vi "Main.vi"(8 "error in":errorcluster, 11 "_Rename in":refnum<class "_Rename.lvclass">) -> (0 "error out":errorcluster, 3 "_Rename out":refnum<class "_Rename.lvclass">)   [LabVIEW 2020, in "_Rename.lvlib" / "_Rename.lvclass"]
uses:
  _Rename.lvclass
  _Rename.lvclass/_Rename.ctl
  _Shared/Project Stuff/Project Stuff.lvclass
  _Shared/Name Specs/Name Specs.lvclass
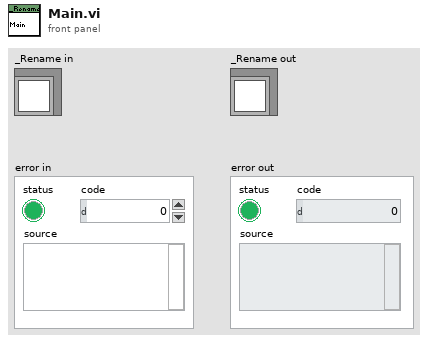
[diagram p1: front panel]
types:
  T1 = typedef "_Shared.lvlib/Name Stuff.ctl" = cluster{"Type (Enum)":T2, "Type (String)":string, "Name Library File Path":path, "Name":string, "Name Type":string}
  T2 = typedef "_Shared.lvlib/Type.ctl" = enum16{"Actor", "Msg"}
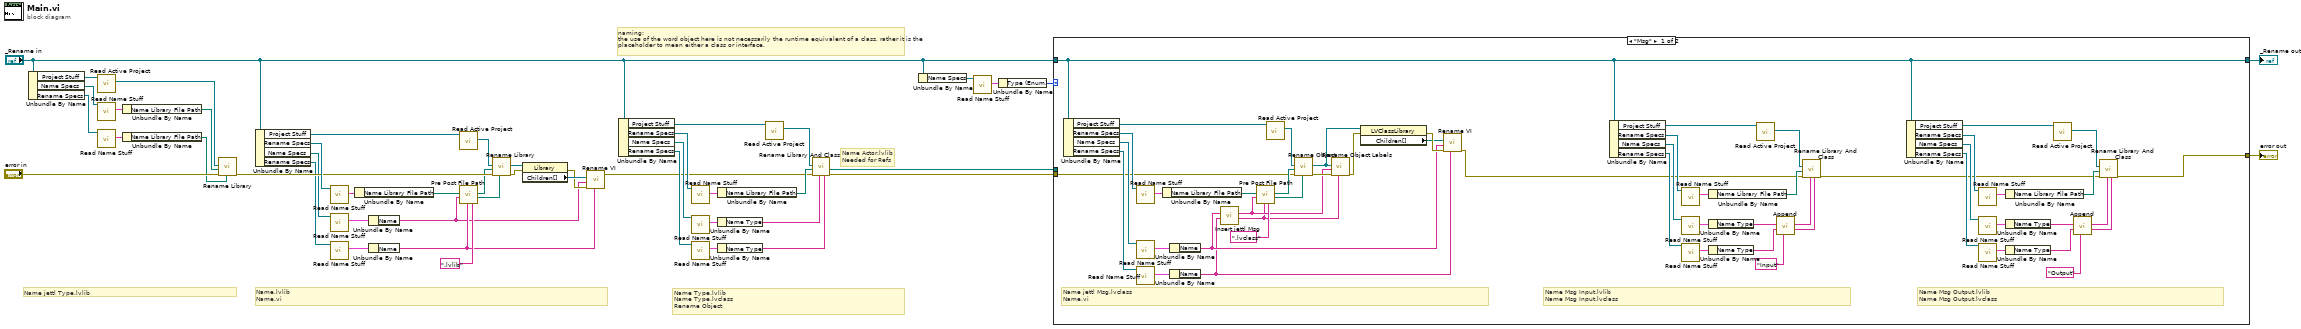
[diagram p0: block diagram]
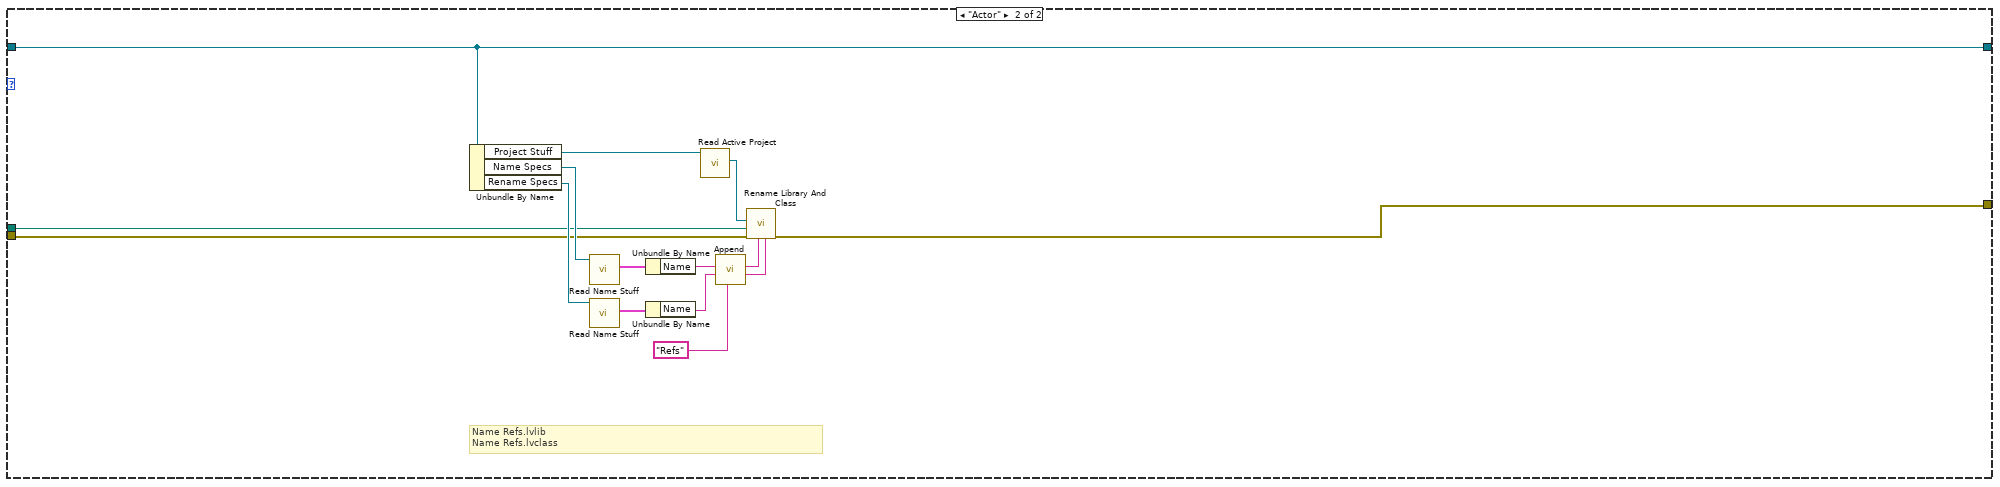
[diagram p2: hidden frame]
diagram:
  # "Name Actor.lvlib\nNeeded for Refs"
  # "Name Type.lvlib\nName Type.lvclass\nRename Object"
  # "naming:\nthe use of the word object here is not necessarily the runtime equivalent of a class, rather it is the placeholder to mean either a class or interface."
  # "Name.lvlib\nName.vi"
  # "Name jettl Type.lvlib"
  n1 = Unbundle By Name("_Rename in") -> ("Project Stuff"=w43:refnum<class "Project Stuff.lvclass">, "Name Specs"=w42:refnum<class "Name Specs.lvclass">, "Rename Specs"=w39:refnum<class "Name Specs.lvclass">)
  n2 = call "Read Active Project.vi"("Project Stuff in"=w43) -> ("Active Project"=w45:refnum<vi>)  [unwired: 10 in]
  n3 = call "Read Name Stuff.vi"("Name Specs in"=w42) -> ("Name Stuff"=w41:T1)  [unwired: 10 in]
  n4 = call "Read Name Stuff.vi"("Name Specs in"=w39) -> ("Name Stuff"=w40:T1)  [unwired: 10 in]
  n5 = Unbundle By Name(w41) -> ("Name Library File Path"=w37:path)
  n6 = Unbundle By Name(w40) -> ("Name Library File Path"=w38:path)
  n7 = call "Rename Library.vi"("Rename Library File Path"=w38, "error in"="error in", "Name Library File Path"=w37, "Active Project"=w45) -> ("error out"=w23:errorcluster)  [unwired: 6 in, 1 out]
  n8 = Unbundle By Name("_Rename in") -> ("Project Stuff"=w25:refnum<class "Project Stuff.lvclass">, "Rename Specs"=w27:refnum<class "Name Specs.lvclass">, "Name Specs"=w21:refnum<class "Name Specs.lvclass">, "Rename Specs"=w18:refnum<class "Name Specs.lvclass">)
  n9 = call "Read Name Stuff.vi"("Name Specs in"=w27) -> ("Name Stuff"=w26:T1)  [unwired: 10 in]
  n10 = call "Read Name Stuff.vi"("Name Specs in"=w21) -> ("Name Stuff"=w20:T1)  [unwired: 10 in]
  n11 = call "Read Name Stuff.vi"("Name Specs in"=w18) -> ("Name Stuff"=w19:T1)  [unwired: 10 in]
  n12 = Unbundle By Name(w26) -> ("Name Library File Path"=w10:path)
  n13 = Unbundle By Name(w20) -> ("Name"=w11:string)
  n14 = Unbundle By Name(w19) -> ("Name"=w12:string)
  n15 = call "Read Active Project.vi"("Project Stuff in"=w25) -> ("Active Project"=w24:refnum<vi>)  [unwired: 10 in]
  n16 = call "Pre Post File Path.vi"("Extension"=".lvlib" ("string"), "Post"=w12, "Pre"=w11, "Rename Library File Path"=w10) -> ("Post File Path"=w8:path, "Pre File Path"=w9:path)  [unwired: 6 in]
  n17 = call "Rename Library.vi"("Rename Library File Path"=w8, "error in"=w23, "Name Library File Path"=w9, "Active Project"=w24) -> ("error out"=w15:errorcluster, "Library Ref"=w17:refnum<vi>)  [unwired: 6 in]
  n18 = property class="Library"(reference=w17, error in=w15) -> (error out=w14:errorcluster, "Children[]"=w16:refnum<vi>[])  [unwired: 1 out]
  n19 = call "Rename VI.vi"("Rename"=w12, "error in"=w14, "VI Name"=w11, "Owned Items[]"=w16) -> ("error out"=w3:errorcluster)  [unwired: 7 in]
  n20 = Unbundle By Name("_Rename in") -> ("Project Stuff"=w44:refnum<class "Project Stuff.lvclass">, "Rename Specs"=w28:refnum<class "Name Specs.lvclass">, "Name Specs"=w29:refnum<class "Name Specs.lvclass">, "Rename Specs"=w30:refnum<class "Name Specs.lvclass">)
  n21 = call "Read Name Stuff.vi"("Name Specs in"=w28) -> ("Name Stuff"=w31:T1)  [unwired: 10 in]
  n22 = call "Read Name Stuff.vi"("Name Specs in"=w29) -> ("Name Stuff"=w33:T1)  [unwired: 10 in]
  n23 = call "Read Name Stuff.vi"("Name Specs in"=w30) -> ("Name Stuff"=w32:T1)  [unwired: 10 in]
  n24 = Unbundle By Name(w31) -> ("Name Library File Path"=w4:path)
  n25 = Unbundle By Name(w33) -> ("Name Type"=w2:string)
  n26 = Unbundle By Name(w32) -> ("Name Type"=w1:string)
  n27 = call "Read Active Project.vi"("Project Stuff in"=w44) -> ("Active Project"=w5:refnum<vi>)  [unwired: 10 in]
  n28 = call "Rename Library And Class.vi"("Post"=w1, "Pre"=w2, "error in"=w3, "Rename Library File Path"=w4, "Active Project"=w5) -> ("error out"=w7:errorcluster, "Intermediate Library File Path"=w6:path)  [unwired: 5 in]
  n29 = Unbundle By Name("_Rename in") -> ("Name Specs"=w34:refnum<class "Name Specs.lvclass">)
  n30 = call "Read Name Stuff.vi"("Name Specs in"=w34) -> ("Name Stuff"=w36:T1)  [unwired: 10 in]
  n31 = Unbundle By Name(w36) -> ("Type (Enum)"=w35:T2)
  n32 = case shown="\"Msg\"" w35 {
    tunnel: w7 -> [w89 w108]
    tunnel: [w53 w103] -> w47
    tunnel: [w55 w112] -> w48
    tunnel: "_Rename in" -> [w55 w112]
    tunnel: w6 -> [_ w106]
    frame "Msg" {
      # "Name Msg Input.lvlib\nName Msg Input.lvclass"
      # "Name Msg Output.lvlib\nName Msg Output.lvclass"
      # "Name jettl Msg.lvclass\nName.vi"
      n33 = Unbundle By Name(w55) -> ("Project Stuff"=w100:refnum<class "Project Stuff.lvclass">, "Rename Specs"=w90:refnum<class "Name Specs.lvclass">, "Name Specs"=w91:refnum<class "Name Specs.lvclass">, "Rename Specs"=w92:refnum<class "Name Specs.lvclass">)
      n34 = call "Read Name Stuff.vi"("Name Specs in"=w90) -> ("Name Stuff"=w94:T1)  [unwired: 10 in]
      n35 = call "Read Name Stuff.vi"("Name Specs in"=w91) -> ("Name Stuff"=w96:T1)  [unwired: 10 in]
      n36 = call "Read Name Stuff.vi"("Name Specs in"=w92) -> ("Name Stuff"=w95:T1)  [unwired: 10 in]
      n37 = Unbundle By Name(w94) -> ("Name Library File Path"=w93:path)
      n38 = Unbundle By Name(w96) -> ("Name"=w52:string)
      n39 = Unbundle By Name(w95) -> ("Name"=w51:string)
      n40 = call "Insert jettl Msg.vi"("Rename"=w51, "Name"=w52) -> ("Post"=w49:string, "Pre"=w50:string)  [unwired: 8 in]
      n41 = call "Pre Post File Path.vi"("Extension"=".lvclass", "Post"=w49, "Pre"=w50, "Rename Library File Path"=w93) -> ("Post File Path"=w98:path, "Pre File Path"=w97:path)  [unwired: 6 in]
      n42 = call "Read Active Project.vi"("Project Stuff in"=w100) -> ("Active Project"=w99:refnum<vi>)  [unwired: 10 in]
      n43 = call "Rename Object.vi"("Post Object File Path"=w98, "error in"=w89, "Pre Object File Path"=w97, "Active Project"=w99) -> ("error out"=w101:errorcluster, "Object Ref"=w88:refnum<vi>)  [unwired: 6 in]
      n44 = call "Rename Object Labels.vi"("Post"=w49, "error in"=w101, "Pre"=w50, "Class Ref"=w88) -> ("error out"=w87:errorcluster)  [unwired: 7 in]
      n45 = property class="LVClassLibrary"(reference=w88, error in=w87) -> (error out=w102:errorcluster, "Children[]"=w86:refnum<vi>[])  [unwired: 1 out]
      n46 = call "Rename VI.vi"("Rename"=w51, "error in"=w102, "VI Name"=w52, "Owned Items[]"=w86) -> ("error out"=w70:errorcluster)  [unwired: 7 in]
      n47 = Unbundle By Name(w55) -> ("Project Stuff"=w84:refnum<class "Project Stuff.lvclass">, "Rename Specs"=w78:refnum<class "Name Specs.lvclass">, "Name Specs"=w79:refnum<class "Name Specs.lvclass">, "Rename Specs"=w80:refnum<class "Name Specs.lvclass">)
      n48 = call "Read Name Stuff.vi"("Name Specs in"=w78) -> ("Name Stuff"=w81:T1)  [unwired: 10 in]
      n49 = call "Read Name Stuff.vi"("Name Specs in"=w79) -> ("Name Stuff"=w83:T1)  [unwired: 10 in]
      n50 = call "Read Name Stuff.vi"("Name Specs in"=w80) -> ("Name Stuff"=w82:T1)  [unwired: 10 in]
      n51 = Unbundle By Name(w81) -> ("Name Library File Path"=w76:path)
      n52 = Unbundle By Name(w83) -> ("Name Type"=w75:string)
      n53 = Unbundle By Name(w82) -> ("Name Type"=w74:string)
      n54 = call "Read Active Project.vi"("Project Stuff in"=w84) -> ("Active Project"=w77:refnum<vi>)  [unwired: 10 in]
      n55 = call "Append.vi"("Append"="Input", "Rename Suffix"=w74, "Name Suffix"=w75) -> ("Post"=w73:string, "Pre"=w72:string)  [unwired: 7 in]
      n56 = call "Rename Library And Class.vi"("Post"=w73, "Pre"=w72, "error in"=w70, "Rename Library File Path"=w76, "Active Project"=w77) -> ("error out"=w54:errorcluster)  [unwired: 5 in, 1 out]
      n57 = Unbundle By Name(w55) -> ("Project Stuff"=w69:refnum<class "Project Stuff.lvclass">, "Rename Specs"=w63:refnum<class "Name Specs.lvclass">, "Name Specs"=w64:refnum<class "Name Specs.lvclass">, "Rename Specs"=w65:refnum<class "Name Specs.lvclass">)
      n58 = call "Read Name Stuff.vi"("Name Specs in"=w63) -> ("Name Stuff"=w66:T1)  [unwired: 10 in]
      n59 = call "Read Name Stuff.vi"("Name Specs in"=w64) -> ("Name Stuff"=w68:T1)  [unwired: 10 in]
      n60 = call "Read Name Stuff.vi"("Name Specs in"=w65) -> ("Name Stuff"=w67:T1)  [unwired: 10 in]
      n61 = Unbundle By Name(w66) -> ("Name Library File Path"=w61:path)
      n62 = Unbundle By Name(w68) -> ("Name Type"=w60:string)
      n63 = Unbundle By Name(w67) -> ("Name Type"=w59:string)
      n64 = call "Read Active Project.vi"("Project Stuff in"=w69) -> ("Active Project"=w62:refnum<vi>)  [unwired: 10 in]
      n65 = call "Append.vi"("Append"="Output", "Rename Suffix"=w59, "Name Suffix"=w60) -> ("Post"=w58:string, "Pre"=w57:string)  [unwired: 7 in]
      n66 = call "Rename Library And Class.vi"("Post"=w58, "Pre"=w57, "error in"=w54, "Rename Library File Path"=w61, "Active Project"=w62) -> ("error out"=w53:errorcluster)  [unwired: 5 in, 1 out]
    }
    frame "Actor" {
      # "Name Refs.lvlib\nName Refs.lvclass"
      n67 = Unbundle By Name(w112) -> ("Project Stuff"=w117:refnum<class "Project Stuff.lvclass">, "Name Specs"=w113:refnum<class "Name Specs.lvclass">, "Rename Specs"=w114:refnum<class "Name Specs.lvclass">)
      n68 = call "Read Name Stuff.vi"("Name Specs in"=w113) -> ("Name Stuff"=w116:T1)  [unwired: 10 in]
      n69 = call "Read Name Stuff.vi"("Name Specs in"=w114) -> ("Name Stuff"=w115:T1)  [unwired: 10 in]
      n70 = Unbundle By Name(w116) -> ("Name"=w110:string)
      n71 = Unbundle By Name(w115) -> ("Name"=w109:string)
      n72 = call "Read Active Project.vi"("Project Stuff in"=w117) -> ("Active Project"=w107:refnum<vi>)  [unwired: 10 in]
      n73 = call "Append.vi"("Append"="Refs" ("input 6"), "Rename Suffix"=w109, "Name Suffix"=w110) -> ("Post"=w104:string, "Pre"=w105:string)  [unwired: 7 in]
      n74 = call "Rename Library And Class.vi"("Post"=w104, "Pre"=w105, "error in"=w108, "Rename Library File Path"=w106, "Active Project"=w107) -> ("error out"=w103:errorcluster)  [unwired: 5 in, 1 out]
    }
  }
  "_Rename out" <- w48
  "error out" <- w47
